vi "STM Basic Server Example.vi"() -> ()   [LabVIEW 2010]
doc: "This example demonstrates how to implement a STM server which sends messages to the client.\n\nThe server needs to be started before the client."
uses:
  vi.lib/NI/STM/SubVIs/MetaDataElement.ctl
  vi.lib/NI/STM/TCP/Write Meta Data (TCP Ref).vi
  vi.lib/NI/STM/TCP/Get Connection Reference (TCP).vi
  vi.lib/NI/STM/TCP/Write Meta Data (TCP Clst).vi
  vi.lib/NI/STM/TCP/Write Message (TCP).vi
  vi.lib/NI/STM/NI STM.lvlib
panel:
  out "error out":errorcluster
  in  "stop":bool
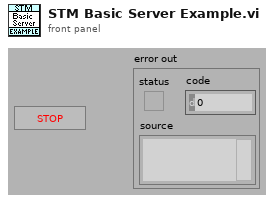
[diagram p1: front panel]
types:
  T1 = typedef "NI STM.lvlib/MetaDataElement.ctl" = string
  T2 = typedef "NI STM.lvlib/TCP Connection Info.ctl" = cluster{"connection ID":refnum<k5>, "meta data":T1[]}
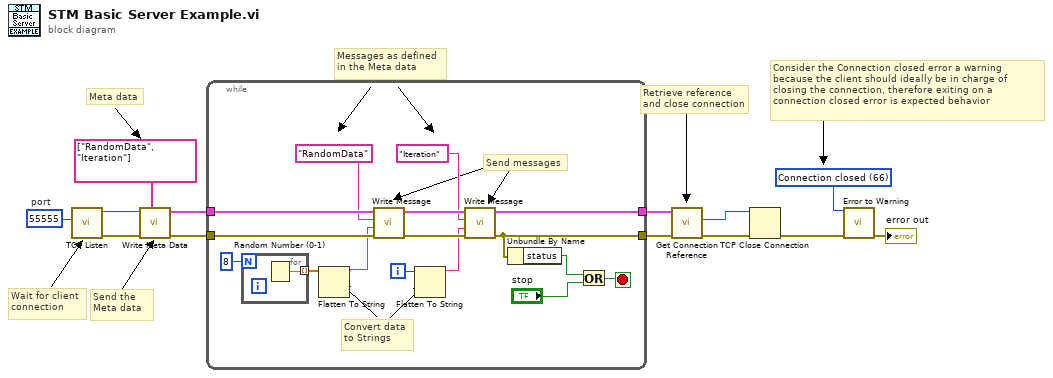
[diagram p0: block diagram]
diagram:
  w4 = 66 items=["No Error", "Argument Error", "Memory Full", "Out of Zone", "End of File", "File Already Open", "Generic File IO Error", "File Not Found", "File Permission Error", "Disk Full", "Duplicate Path", "Too Many Files Open", "Not Enabled", "Resource File Not Found", "Cannot Add Resource", "Resource Not Found", "Image Not Found", "Image Memory Error", "Pen Does Not Exist", "Config Bad Type", "Config Token Not Found", "Config Parse Error", "Config Memory Error", "Bad External Code Format", "Bad External Code Offset", "External Code Not Present", "Null Window", "Destroy Window Mixup", "Null Menu", "Print Aborted", "Bad Print Record", "Print Driver Error", "Windows Error During Print", "Memory Error During Print", "Print Dialog Error", "Generic Print Error", "Invalid Device Refnum", "Device Not Found", "Device Parameter Error", "Device Unit Error", "Can't Open Device", "Device Call Aborted", "Generic Error", "Cancelled By User", "Object ID Too Low", "Object ID Too High", "Object Not In Heap", "Unknown Heap", "Bad DefProc ID", "DefProc Not In Table", "Message Out Of Range", "Null Method", "Unknown Message", "Manager Call Not Supported", "Bad address", "Connection In progress", "Connection timed out", "Connection is already in progress", "Network attribute not supported", "Network error", "Address in use", "System out of memory", "Connection aborted", "Connection refused", "Connection is not connected", "Connection is already connected", "Connection closed", "Initialize error (interapplication manager)", "Bad occurrence", "Wait on unbound occurrence handler", "Occurrence queue overflow", "Bad path", "Semaphore not signaled", "Unrecognized type (interapplication manager)"] ("1st Error to Convert")
  w13 = u16 55555  # port
  # "Consider the Connection closed error a warning because the client should ideally be in charge of closing the connection, therefore exiting on a connection closed error is expected behavior"
  # "Retrieve reference and close connection"
  # "Meta data"
  # "Messages as defined\nin the Meta data"
  # "Wait for client\nconnection"
  # "Send the\nMeta data"
  n1 = call <vilib>:"TCP Listen.vi"("port"=w13) -> ("error out"=w11:errorcluster, "connection ID"=w12:refnum<k5>)  [unwired: 3 in, 6 out]
  n2 = call-poly "Write Meta Data.vi"("meta data"=T1[] ["RandomData", "Iteration"] ("Meta data"), "error in"=w11, "connection ID"=w12) -> ("error out"=w9:errorcluster, "connection info out"=w10:T2)  [unwired: 2 in, 5 out]
  n3 = while {
    tunnel: w10 -> [w29]
    tunnel: w9 -> [w28]
    tunnel: [w27] -> w8
    tunnel: [w20] -> w6
    i -> [w15]
    stop <- w21 stop-if-true
    # "Send messages"
    # "Convert data\nto Strings"
    n4 = for {
      N: 8 -> [_]
      tunnel: [w30] -> w17 mode=indexing
      n5 = Random Number (0-1)() -> (number: 0 to 1=w30:dbl)
    }
    n6 = Flatten To String(anything=w17) -> (data string=w16:string)  [unwired: 1 in, 4 out]
    n7 = call-poly "Write Message.vi"("error in"=w28, "data"=w16, "name"="RandomData" ("Name"), "connection info in"=w29) -> ("error out"=w26:errorcluster, "connection info out"=w25:T2)  [unwired: 1 in, 5 out]
    n8 = Flatten To String(anything=w15) -> (data string=w14:string)  [unwired: 1 in, 4 out]
    n9 = call-poly "Write Message.vi"("error in"=w26, "data"=w14, "name"="Iteration" ("Name"), "connection info in"=w25) -> ("error out"=w20:errorcluster, "connection info out"=w27:T2)  [unwired: 1 in, 5 out]
    n10 = Unbundle By Name(w20) -> ("status"=w19:bool)
    n11 = Or(x=w19, y="stop") -> (x .or. y?=w21:bool)
  }
  n12 = call-poly "Get Connection Reference.vi"("error in"=w6, "connection info in"=w8) -> ("error out"=w5:errorcluster, "connection ID out"=w7:refnum<k5>)  [unwired: 8 out]
  n13 = TCP Close Connection(connection ID=w7, error in (no error)=w5) -> (error out=w3:errorcluster)  [unwired: 2 out]
  n14 = call <vilib>:"Error to Warning.vi"("1st Error to Convert"=w4, "error in"=w3) -> ("warning out"=→"error out":errorcluster)  [unwired: 3 in, 10 out]
